vi "pulse shaping filter.vi"() -> ()   [LabVIEW 2018]
panel:
  in  "IQ symbols":cdb[](array[numeric])
  in  "filter parameter":dbl=0.5 format="%.2f"
  out "IQ pulses":cdb[](array[numeric])
  in  "modulation type":T1(ring)
  in  "pulse shaping samples per symbol (16)":i32=16
  in  "pulse shaping filter (none)":T2(ring)
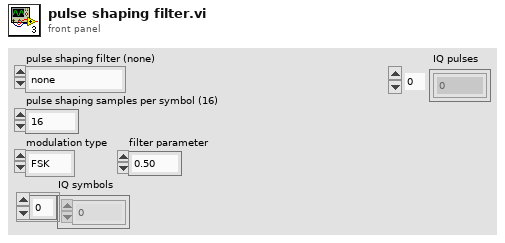
[diagram p1: front panel]
types:
  T1 = enum16{"FSK", "PSK", "QAM", "MSK", "PAM", "ASK", "CPM"}
  T2 = enum16{"none", "Raised Cosine", "Root Raised Cos", "Gaussian"}
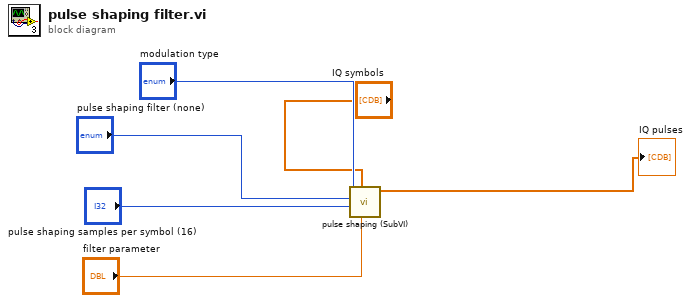
[diagram p0: block diagram]
diagram:
  n1 = call "pulse shaping (SubVI).vi"("filter parameter"="filter parameter", "IQ symbols"="IQ symbols", "pulse shaping samples per symbol (16)"="pulse shaping samples per symbol (16)", "pulse shaping filter (none)"="pulse shaping filter (none)", "modulation type"="modulation type") -> ("X * Y"=→"IQ pulses":cdb[])  [unwired: 6 in]
